vi "Read InformIgor.vi"(8 "error in (no error)":errorcluster, 11 "Variable in":refnum<class "Variable.lvclass">) -> (0 "error out":errorcluster, 2 "InformIgor":bool, 3 "Variable out":refnum<class "Variable.lvclass">)   [LabVIEW 2013, in "Variable.lvclass"]
uses:
  Variable.lvclass
  Variable.lvclass/Variable.ctl
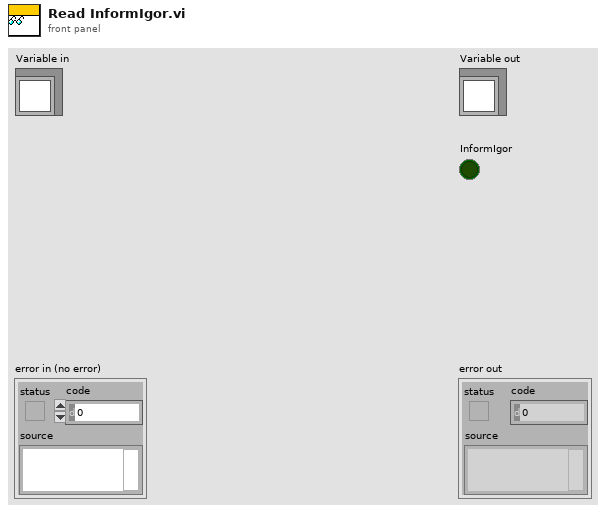
[diagram p1: front panel]
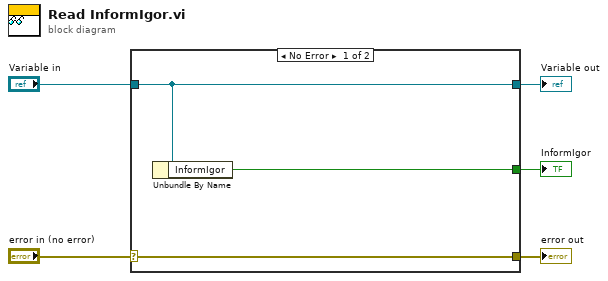
[diagram p0: block diagram]
diagram:
  n1 = case shown="No Error" "error in (no error)" {
    selector: "error in (no error)" -> [w8 w9]
    tunnel: [w8 w9] -> w4
    tunnel: [w7 w10] -> w2
    tunnel: "Variable in" -> [w7 w10]
    tunnel: [w6 _] -> w1
    frame No Error {
      n2 = Unbundle By Name(w7) -> ("InformIgor"=w6:bool)
    }
    frame Error {
    }
  }
  "error out" <- w4
  "Variable out" <- w2
  "InformIgor" <- w1
